vi "Pololu.Dual Servo Parse Args for Funct Move.vi"(11 "Args":string[](array[string])) -> (3 "Params":T1)   [LabVIEW 2018]
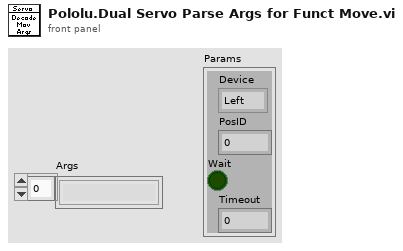
[diagram p1: front panel]
types:
  T1 = cluster{"Device":enum16{"Left", "Right", "All"}, "PosID":u8, "Wait":bool, "Timeout":dbl}
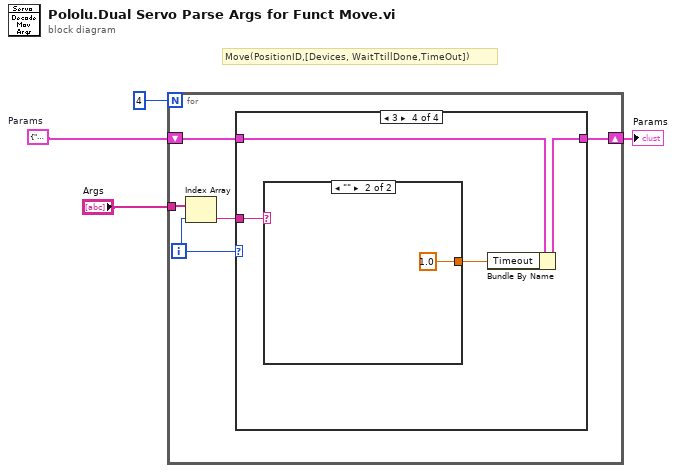
[diagram p0: block diagram]
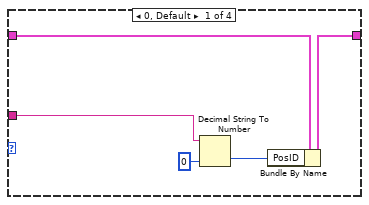
[diagram p2: hidden frame]
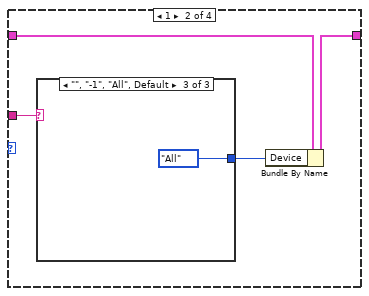
[diagram p3: hidden frame]
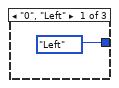
[diagram p4: hidden frame]
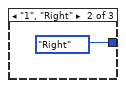
[diagram p5: hidden frame]
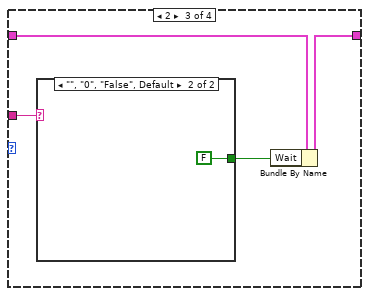
[diagram p6: hidden frame]
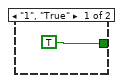
[diagram p7: hidden frame]
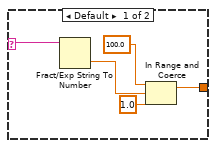
[diagram p8: hidden frame]
diagram:
  w2 = T1 {"Device"=enum."Left", "PosID"=0, "Wait"=FALSE, "Timeout"=0.0}  # Params
  # "Move(PositionID,[Devices, WaitTtillDone,TimeOut])"
  n1 = for {
    N: 4 -> [_]
    tunnel: "Args" -> [w9]
    shift-right: [w5] -> w1
    shift-left: w2 -> [w6]
    i -> [w8]
    n2 = Index Array(array=w9, index=w8) -> (element=w7:string)
    n3 = case shown="3" w8 {
      tunnel: w7 -> [w12 w16 w23 w29]
      tunnel: w6 -> [w14 w18 w25 w31]
      tunnel: [w13 w17 w24 w30] -> w5
      frame 0, Default {
        n4 = Decimal String To Number(string=w12, default (0L)=u8 0 ("default (0 I32)")) -> (number=w11:u8)  [unwired: 1 in, 1 out]
        n5 = Bundle By Name(cluster=w14, "PosID"=w11) -> (w13:T1)
      }
      frame 1 {
        n6 = case shown="\"\", \"-1\", \"All\", Default" w16 {
          tunnel: [enum16{"Left", "Right", "All"}."Left" ("Device") enum16{"Left", "Right", "All"}."Right" ("Device") enum16{"Left", "Right", "All"}."All" ("Device")] -> w15
          frame "0", "Left" {
          }
          frame "1", "Right" {
          }
          frame "", "-1", "All", Default {
          }
        }
        n7 = Bundle By Name(cluster=w18, "Device"=w15) -> (w17:T1)
      }
      frame 2 {
        n8 = case shown="\"\", \"0\", \"False\", Default" w23 {
          tunnel: [TRUE FALSE] -> w22
          frame "1", "True" {
          }
          frame "", "0", "False", Default {
          }
        }
        n9 = Bundle By Name(cluster=w25, "Wait"=w22) -> (w24:T1)
      }
      frame 3 {
        n10 = case shown="\"\"" w29 {
          selector: w29 -> [w35 _]
          tunnel: [w36 1.0] -> w28
          frame Default {
            n11 = Fract/Exp String To Number(string=w35) -> (number=w34:dbl)  [unwired: 3 in, 1 out]
            n12 = In Range and Coerce(upper limit=100.0, x=w34, lower limit=1.0) -> (coerced(x)=w36:dbl)  [unwired: 1 out]
          }
          frame "" {
          }
        }
        n13 = Bundle By Name(cluster=w31, "Timeout"=w28) -> (w30:T1)
      }
    }
  }
  "Params" <- w1
